vi "Open_Redis.vi"(0 "Host":string="localhost", 5 "Port":u16=6379, 11 "error in":errorcluster) -> (4 "Refnum out":refnum<vi>, 8 "Connection ok ?":bool, 15 "error out":errorcluster)   [LabVIEW 2023]
uses:
  Redis Commands/Connection/PING.vi
panel:
  out "output cluster":cluster{"host":string, "port":u16}
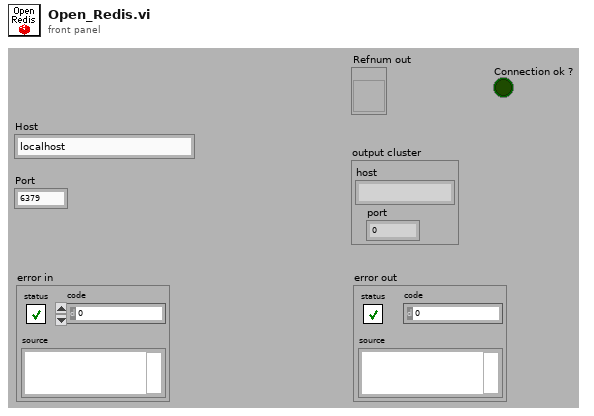
[diagram p1: front panel]
types:
  T1 = enum16{"None", "Error", "Status", "Nil", "Integer", "String", "Multibulk"}
  T2 = typedef "redis-data.ctl" = cluster{"type":enum16{"None", "Error", "Status", "Nil", "Integer", "String", "Multibulk"}, "integer":i64, "string":string, "multibulk":variant[], "string data":string[]}
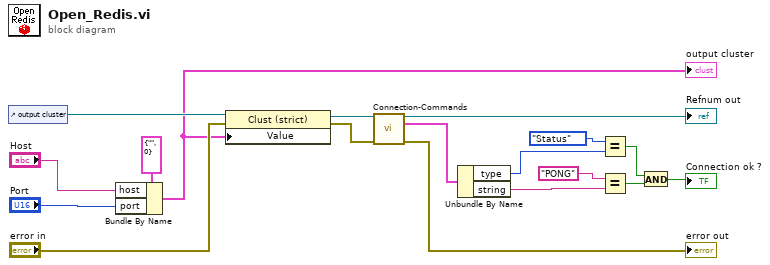
[diagram p0: block diagram]
diagram:
  n1 = control-ref of="output cluster"() -> (w14:refnum<vi>)
  n2 = Bundle By Name(cluster=cluster{"host":string, "port":u16} {"host"="", "port"=0} ("Value"), "host"="Host", "port"="Port") -> (w1:cluster{"host":string, "port":u16})
  "output cluster" <- w1
  n3 = property class="Clust (strict)"(reference=w14, error in="error in", "Value"=w1) -> (reference out=w13:refnum<vi>, error out=w12:errorcluster)
  n4 = call-poly "Connection-Commands.vi"("refnum in"=w13, "error in"=w12) -> ("refnum out"=→"Refnum out":refnum<vi>, "Data"=w4:T2, "error out"=→"error out":errorcluster)  [unwired: 11 in]
  n5 = Unbundle By Name(w4) -> ("type"=w3:T1, "string"=w6:string)
  n6 = Equal?(x=T1."Status" ("type"), y=w3) -> (x = y?=w9:bool)
  n7 = Equal?(x="PONG", y=w6) -> (x = y?=w8:bool)
  n8 = And(x=w9, y=w8) -> (x .and. y?=→"Connection ok ?":bool)
